vi "Capture_Save_Initialize.vi"(11 "input cluster":T1={"L16 Linear Actuator"="", "XE 1000 Pump"="", "Camera1"="", "Camera2"="", "Camera1_IMG"=refnum, "Camera2_IMG"=refnum, "Img_Capt"=FALSE, "Actuator"=FALSE, "Pump"=FALSE, "Cam 1"=FALSE, "Cam 2"=FALSE, "Empty_Refill"=FALSE, "Crop"=FALSE, "Light intensity"=100, "Exposure Time"=1000.0, "Sample Name"="Test Sample", "Operator"="MRJ", "Calibration 1"=path "C:/Users/au540322/Desktop/IHS_Project/images/Debris/Debris_0/Debris_0_2019_06_01-23-32-49-686.PNG", "Calibration 2"=path "C:/Users/au540322/Desktop/IHS_Project/images/Debris/Debris_0/Debris_0_2019_06_01-23-32-49-686.PNG", "Framerate"=1, "Timeout Sample"=200, "Collection date"="", "Sample size threshold"=1, "Empty start"=1, "Command"="MRJ", "Calibration Image 1"=refnum, "Calibration Image 2"=refnum, "Original Image 1"=refnum, "Original Image 2"=refnum, "Processing Image 1"=refnum, "Processing Image 2"=refnum, "Object Image 1"=refnum, "Object Image 2"=refnum, "Cam 1 - save queue"=refnum, "Cam 2 - save queue"=refnum, "Station"="", "Species Name"="", "Other Notes"="", "Aperture"=enum."Item 0", "Image Process Queue Size"=500, "Image Save Queue Size"=500, "Overload threshold"=500, "Max Framerate"=100, "Blue Plane Image"=refnum, "Subtract Image"=refnum, "Binary Image 1"=refnum, "ROI mask allocation"=refnum, "Rectangle 1"={"Left"=0, "Top"=0, "Right"=0, "Bottom"=0, "Rotation"=0.0}, "Rectangle 2"={"Left"=0, "Top"=0, "Right"=0, "Bottom"=0, "Rotation"=0.0}, "Binary Image 2"=refnum, "Detection Region %"=0.0, "Cam 1 queue"=refnum, "Cam 2 queue"=refnum, "Detect image 1"=refnum, "Detect image 2"=refnum, "Detect 1"=path "C:/Users/au540322/Desktop/IHS_Project/images/Debris/Debris_0/Debris_0_2019_06_01-23-32-49-686.PNG", "Detect 2"=path "C:/Users/au540322/Desktop/IHS_Project/images/Debris/Debris_0/Debris_0_2019_06_01-23-32-49-686.PNG", "Max large object threshold"=0, "Open(T)/Close(F)"=FALSE} {"Rectangle 2"."Rotation" format="%.2f"; "Rectangle 2"."Left" scale=0.0..1024.0; "Rectangle 2"."Right" scale=0.0..1024.0; "Rectangle 1"."Rotation" format="%.2f"; "Rectangle 1"."Left" scale=0.0..1024.0; "Rectangle 1"."Right" scale=0.0..1024.0; "Max Framerate" min=1; "Overload threshold" min=1; "Image Save Queue Size" min=1; "Image Process Queue Size" min=1; "Empty start" min=1; "Sample size threshold" min=1; "Framerate" min=1; "Light intensity" scale=0.0..100.0}) -> (3 "output cluster":T1={"L16 Linear Actuator"="", "XE 1000 Pump"="", "Camera1"="", "Camera2"="", "Camera1_IMG"=refnum, "Camera2_IMG"=refnum, "Img_Capt"=FALSE, "Actuator"=FALSE, "Pump"=FALSE, "Cam 1"=FALSE, "Cam 2"=FALSE, "Empty_Refill"=FALSE, "Crop"=FALSE, "Light intensity"=100, "Exposure Time"=1000.0, "Sample Name"="Test Sample", "Operator"="MRJ", "Calibration 1"=path "C:/Users/au540322/Desktop/IHS_Project/images/Debris/Debris_0/Debris_0_2019_06_01-23-32-49-686.PNG", "Calibration 2"=path "C:/Users/au540322/Desktop/IHS_Project/images/Debris/Debris_0/Debris_0_2019_06_01-23-32-49-686.PNG", "Framerate"=100, "Timeout Sample"=200, "Collection date"="", "Sample size threshold"=500, "Empty start"=1, "Command"="", "Calibration Image 1"=refnum, "Calibration Image 2"=refnum, "Original Image 1"=refnum, "Original Image 2"=refnum, "Processing Image 1"=refnum, "Processing Image 2"=refnum, "Object Image 1"=refnum, "Object Image 2"=refnum, "Cam 1 - save queue"=refnum, "Cam 2 - save queue"=refnum, "Station"="", "Species Name"="", "Other Notes"="", "Aperture"=enum."Item 0", "Image Process Queue Size"=500, "Image Save Queue Size"=500, "Overload threshold"=500, "Max Framerate"=100, "Blue Plane Image"=refnum, "Subtract Image"=refnum, "Binary Image 1"=refnum, "ROI mask allocation"=refnum, "Rectangle 1"={"Left"=0, "Top"=0, "Right"=0, "Bottom"=0, "Rotation"=0.0}, "Rectangle 2"={"Left"=0, "Top"=0, "Right"=0, "Bottom"=0, "Rotation"=0.0}, "Binary Image 2"=refnum, "Detection Region %"=0.0, "Cam 1 queue"=refnum, "Cam 2 queue"=refnum, "Detect image 1"=refnum, "Detect image 2"=refnum, "Detect 1"=path "C:/Users/au540322/Desktop/IHS_Project/images/Debris/Debris_0/Debris_0_2019_06_01-23-32-49-686.PNG", "Detect 2"=path "C:/Users/au540322/Desktop/IHS_Project/images/Debris/Debris_0/Debris_0_2019_06_01-23-32-49-686.PNG", "Max large object threshold"=0, "Open(T)/Close(F)"=FALSE} {"Rectangle 2"."Rotation" format="%.2f"; "Rectangle 2"."Left" scale=0.0..1024.0; "Rectangle 2"."Right" scale=0.0..1024.0; "Rectangle 1"."Rotation" format="%.2f"; "Rectangle 1"."Left" scale=0.0..1024.0; "Rectangle 1"."Right" scale=0.0..1024.0; "Max Framerate" min=1; "Overload threshold" min=1; "Image Save Queue Size" min=1; "Image Process Queue Size" min=1; "Empty start" min=1; "Sample size threshold" min=1; "Framerate" min=1; "Light intensity" scale=0.0..100.0})   [LabVIEW 2019]
uses:
  controls/Data.ctl
  <vilib>/userdefined/High Color/IMAQdx.ctl
  <vilib>/vision/Image Controls.llb/IMAQ Image.ctl
  <vilib>/vision/driver/IMAQdx.llb/IMAQdx Acquisition Mode.ctl
  <vilib>/vision/driver/NI_Vision_Acquisition_Software.lvlib
types:
  T1 = typedef "Data.ctl" = cluster{"L16 Linear Actuator":refnum<visa-resource-name>, "XE 1000 Pump":refnum<visa-resource-name>, "Camera1":T2, "Camera2":T2, "Camera1_IMG":T3, "Camera2_IMG":T3, "Img_Capt":bool, "Actuator":bool, "Pump":bool, "Cam 1":bool, "Cam 2":bool, "Empty_Refill":bool, "Crop":bool, "Light intensity":i32, "Exposure Time":dbl, "Sample Name":string, "Operator":string, "Calibration 1":path, "Calibration 2":path, "Framerate":i32, "Timeout Sample":i32, "Collection date":string, "Sample size threshold":i32, "Empty start":u32, "Command":string, "Calibration Image 1":T3, "Calibration Image 2":T3, "Original Image 1":T3, "Original Image 2":T3, "Processing Image 1":T3, "Processing Image 2":T3, "Object Image 1":T3, "Object Image 2":T3, "Cam 1 - save queue":refnum<queue>, "Cam 2 - save queue":refnum<queue>, "Station":string, "Species Name":string, "Other Notes":string, "Aperture":enum32{"Item 0", "Item 1", "Item 2", "Item 3"}, "Image Process Queue Size":i32, "Image Save Queue Size":i32, "Overload threshold":i32, "Max Framerate":i32, "Blue Plane Image":T3, "Subtract Image":T3, "Binary Image 1":T3, "ROI mask allocation":T3, "Rectangle 1":T4, "Rectangle 2":T4, "Binary Image 2":T3, "Detection Region %":dbl, "Cam 1 queue":refnum<queue>, "Cam 2 queue":refnum<queue>, "Detect image 1":T3, "Detect image 2":T3, "Detect 1":path, "Detect 2":path, "Max large object threshold":i32, "Open(T)/Close(F)":bool}
  T2 = typedef "IMAQdx.ctl" = refnum<k21>
  T3 = typedef "IMAQ Image.ctl" = refnum<image>
  T4 = typedef "IMAQ Rectangle" = cluster{"Left":i32, "Top":i32, "Right":i32, "Bottom":i32, "Rotation":dbl}
  T5 = typedef "Image Type" = u32
  T6 = cluster{"Timestamp":string, "Image Pixels (U32)":u32[][], i32}
  T7 = typedef "NI_Vision_Acquisition_Software.lvlib/IMAQdx Acquisition Mode.ctl" = enum32{"One Shot", "Continuous"}
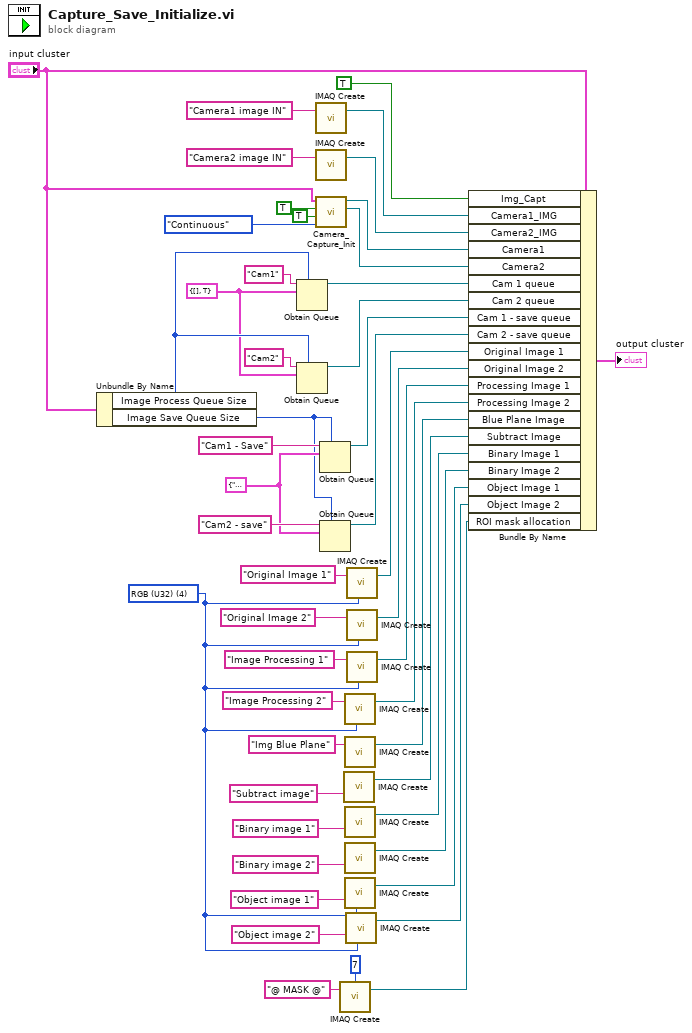
[diagram p0: block diagram]
diagram:
  w1 = cluster{"Image Pixels (U32)":u32[][], bool} {"Image Pixels (U32)"=[], TRUE}
  w8 = T5 4 items=["Grayscale (U8)", "Grayscale (I16)", "Grayscale (SGL)", "Complex (CSG)", "RGB (U32)", "HSL (U32)", "RGB (U64)", "Grayscale (U16)"] ("Image Type")
  w30 = T6 {"Timestamp"="", "Image Pixels (U32)"=[], 0} ("output cluster 2")
  n1 = Unbundle By Name("input cluster") -> ("Image Process Queue Size"=w20:i32, "Image Save Queue Size"=w19:i32)
  n2 = Obtain Queue(max queue size (-1, unlimited)=w20, name (unnamed)="Cam1", element data type=w1) -> (queue out=w38:refnum<queue>)  [unwired: 2 in, 2 out]
  n3 = Obtain Queue(max queue size (-1, unlimited)=w20, name (unnamed)="Cam2", element data type=w1) -> (queue out=w37:refnum<queue>)  [unwired: 2 in, 2 out]
  n4 = call "IMAQ Create"("Image Name"="Camera1 image IN") -> ("New Image"=w46:T3)  [unwired: 4 in, 1 out]
  n5 = call "IMAQ Create"("Image Name"="Camera2 image IN") -> ("New Image"=w45:T3)  [unwired: 4 in, 1 out]
  n6 = call "Camera_Capture_Init.vi"("Continuous?"=IMAQdx_Acquisition_Mode."Continuous", "Detect Movement"=TRUE, "Crop?"=TRUE, "input cluster"="input cluster") -> ("Camera2"=w42:T2, "Camera1"=w43:T2)  [unwired: 6 in]
  n7 = Obtain Queue(max queue size (-1, unlimited)=w19, name (unnamed)="Cam1 - Save", element data type=w30) -> (queue out=w33:refnum<queue>)  [unwired: 2 in, 2 out]
  n8 = Obtain Queue(max queue size (-1, unlimited)=w19, name (unnamed)="Cam2 - save", element data type=w30) -> (queue out=w32:refnum<queue>)  [unwired: 2 in, 2 out]
  n9 = call "IMAQ Create"("Border Size"=7, "Image Name"="@ MASK @") -> ("New Image"=w5:T3)  [unwired: 2 in, 2 out]
  n10 = call "IMAQ Create"("Image Name"="Subtract image") -> ("New Image"=w15:T3)  [unwired: 3 in, 2 out]
  n11 = call "IMAQ Create"("Image Name"="Image Processing 2", "Image Type"=w8) -> ("New Image"=w22:T3)  [unwired: 2 in, 2 out]
  n12 = call "IMAQ Create"("Image Name"="Img Blue Plane") -> ("New Image"=w17:T3)  [unwired: 3 in, 2 out]
  n13 = call "IMAQ Create"("Image Name"="Binary image 1") -> ("New Image"=w13:T3)  [unwired: 3 in, 2 out]
  n14 = call "IMAQ Create"("Image Name"="Binary image 2") -> ("New Image"=w3:T3)  [unwired: 3 in, 2 out]
  n15 = call "IMAQ Create"("Image Name"="Object image 1", "Image Type"=w8) -> ("New Image"=w10:T3)  [unwired: 2 in, 2 out]
  n16 = call "IMAQ Create"("Image Name"="Object image 2", "Image Type"=w8) -> ("New Image"=w9:T3)  [unwired: 2 in, 2 out]
  n17 = call "IMAQ Create"("Image Name"="Original Image 1", "Image Type"=w8) -> ("New Image"=w25:T3)  [unwired: 2 in, 2 out]
  n18 = call "IMAQ Create"("Image Name"="Original Image 2", "Image Type"=w8) -> ("New Image"=w24:T3)  [unwired: 2 in, 2 out]
  n19 = call "IMAQ Create"("Image Name"="Image Processing 1", "Image Type"=w8) -> ("New Image"=w23:T3)  [unwired: 2 in, 2 out]
  n20 = Bundle By Name(cluster="input cluster", "Img_Capt"=TRUE ("Image_Capture"), "Camera1_IMG"=w46, "Camera2_IMG"=w45, "Camera1"=w43, "Camera2"=w42, "Cam 1 queue"=w38, "Cam 2 queue"=w37, "Cam 1 - save queue"=w33, "Cam 2 - save queue"=w32, "Original Image 1"=w25, "Original Image 2"=w24, "Processing Image 1"=w23, "Processing Image 2"=w22, "Blue Plane Image"=w17, "Subtract Image"=w15, "Binary Image 1"=w13, "Binary Image 2"=w3, "Object Image 1"=w10, "Object Image 2"=w9, "ROI mask allocation"=w5) -> (→"output cluster":T1)
